vi "Configure Trigger.vi"(6 "Manual Trigger Delay (5.0 s)":dbl=5.0, 8 "error in (no error)":errorcluster, 9 "Auto Delay (T:Enable)":bool=TRUE, 10 "Trigger Source (0: Immediate)":u16(ring) items=["Immediate", "Software (Bus)", "External"], 11 "VISA resource name":refnum<visa-resource-name>) -> (0 "error out":errorcluster, 3 "VISA resource name out":refnum<visa-resource-name>)   [LabVIEW 2015, in "Template - DMM.lvlib"]
doc: "Configures the trigger settings on the instrument.\n\n<B>Note:</B> Use this VI only with other low-level VIs. The high-level VIs automatically incorporate this functionality."
uses:
  <instrlib>/_Template - DMM/Template - DMM.lvlib
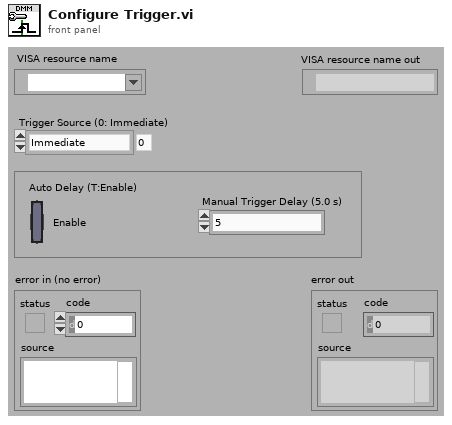
[diagram p1: front panel]
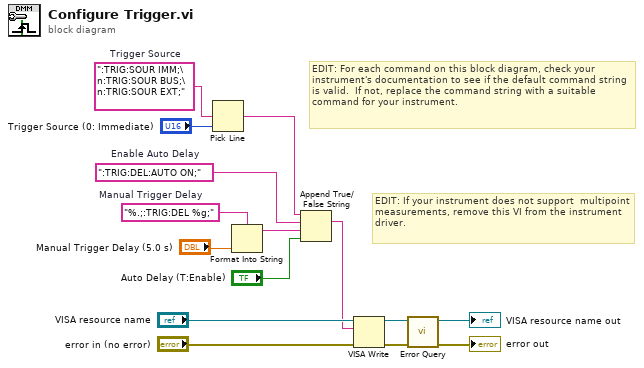
[diagram p0: block diagram]
diagram:
  w4 = ":TRIG:DEL:AUTO ON;"  # Enable Auto Delay
  w5 = "%.;:TRIG:DEL %g;"  # Manual Trigger Delay
  w12 = ":TRIG:SOUR IMM;\n:TRIG:SOUR BUS;\n:TRIG:SOUR EXT;"  # Trigger Source
  # "EDIT: If your instrument does not support  multipoint measurements, remove this VI from the instrument driver."
  # "EDIT: For each command on this block diagram, check your instrument's documentation to see if the default command string is valid.  If not, replace the command string with a suitable command for your instrument."
  n1 = Pick Line(multi-line string=w12, line index="Trigger Source (0: Immediate)") -> (output string=w2:string)  [unwired: 1 in]
  n2 = Format Into String(format string=w5, "Manual Trigger Delay (5.0 s)") -> (resulting string=w3:string)  [unwired: 2 in, 1 out]
  n3 = Append True/False String(1:"Auto Delay (T:Enable)", 2:w3, 3:w4, 4:w2) -> (0:w1:string)
  n4 = VISA Write(VISA resource name="VISA resource name", write buffer=w1, error in (no error)="error in (no error)") -> (VISA resource name out=w9:refnum<visa-resource-name>, error out=w8:errorcluster)  [unwired: 1 out]
  n5 = call <instrlib>:"Error Query.vi"("error in (no error)"=w8, "VISA resource name"=w9) -> ("error out"=→"error out":errorcluster, "VISA resource name out"=→"VISA resource name out":refnum<visa-resource-name>)  [unwired: 6 in, 2 out]
